vi "New JSON (String).vi"(8 "error in (no error)":errorcluster, 10 "value":string) -> (0 "error out":errorcluster, 3 "JSON Value out":refnum<class "JSON Value.lvclass">)   [LabVIEW 2016, in "JSON Value.lvclass"]
doc: "Create a new JSON String with the given value"
uses:
  JSON Value.lvclass
  JSON Types.ctl
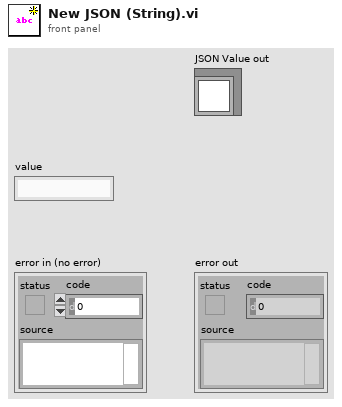
[diagram p1: front panel]
types:
  T1 = typedef "JSON Value.lvclass/JSON Types.ctl" = enum16{"String", "Numeric", "Boolean", "NULL", "Object", "Array"}
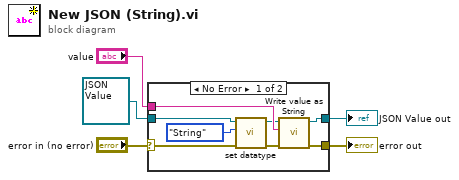
[diagram p0: block diagram]
diagram:
  n1 = case shown="No Error" "error in (no error)" {
    selector: "error in (no error)" -> [w13 w15]
    tunnel: [w10 w15] -> w4
    tunnel: [w11 w14] -> w3
    tunnel: "value" -> [w12 _]
    tunnel: refnum<class "JSON Value.lvclass"> refnum ("JSON out") -> [w8 w14]
    frame No Error {
      n2 = call "set datatype.vi"("error in (no error)"=w13, "datatype"=JSON_Types."String", "JSON Helper in"=w8) -> ("error out"=w9:errorcluster, "JSON Helper out"=w7:refnum<class "JSON Value.lvclass">)  [unwired: 7 in]
      n3 = call "Write value as String.vi"("error in (no error)"=w9, "value"=w12, "JSON Value in"=w7) -> ("error out"=w10:errorcluster, "JSON Value out"=w11:refnum<class "JSON Value.lvclass">)  [unwired: 7 in]
    }
    frame Error {
    }
  }
  "error out" <- w4
  "JSON Value out" <- w3
